vi "Actor Core.vi"(8 "error in":errorcluster, 11 "Philosopher in":refnum<class "Philosopher.lvclass">) -> (0 "error out":errorcluster, 3 "Philosopher out":refnum<class "Actor.lvclass">)   [LabVIEW 2023, in "Philosopher.lvlib" / "Philosopher.lvclass"]
doc: "(<B>Filename</B>: Actor Framework.lvlib:Actor.lvclass:Actor Core.vi)\n\nReceives messages to the actor, reacts to them, and initiates any error handling that may shut the actor down.\n\nDescendant classes may override this VI to append parallel tasks for the actor to complete while it handles messages. Overrides use the Call Parent Method node."
uses:
  Philosopher.lvclass
  C:/Program Files (x86)/National Instruments/LabVIEW 2023/vi.lib/ActorFramework/Actor/Actor.lvclass
  <vilib>/ActorFramework/Actor/Actor.lvclass
  State Picture.ctl
  Philosopher Statechart.lvsc/Inputs.ctl
  <vilib>/ActorFramework/Message Enqueuer/Message Enqueuer.lvclass
  Philosopher Statechart.lvsc/Trigger.ctl
  Philosopher.lvclass/Philosopher.ctl
  <vilib>/ActorFramework/Actor/Actor.lvclass/Actor.ctl
  <vilib>/ActorFramework/Message Enqueuer/Message Enqueuer.lvclass/Message Enqueuer.ctl
  <vilib>/Statechart/Common/IntGuid.ctl
  <vilib>/Statechart/Common/DbgID.ctl
  Philosopher Statechart.lvsc/StatechartState.ctl
  Philosopher Statechart.lvsc/State.ctl
  031f544c-a229-44b1-b513-832e3cf1e2d7.vi
  <vilib>/ActorFramework/Message Enqueuer/Init from Existing Queue.vi
  Philosopher Statechart.lvsc/CompanionDiagram.vi/26/SC Main.vi
  <vilib>/Statechart/Infrastructure/RTStatechart/RunTime SCN.xnode
  Philosopher Statechart.lvsc/Outputs.ctl
  Philosopher Statechart.lvsc
  <vilib>/Statechart/Nodes/EventFiring/NI_SC_EventFiringNode.xnode
  <vilib>/Statechart/Common/NI_SC_LVSCCommonFiles.lvlib
panel:
  out "Diagram Display":picture
  out "ID":i32
  out "State Picture":T1=3
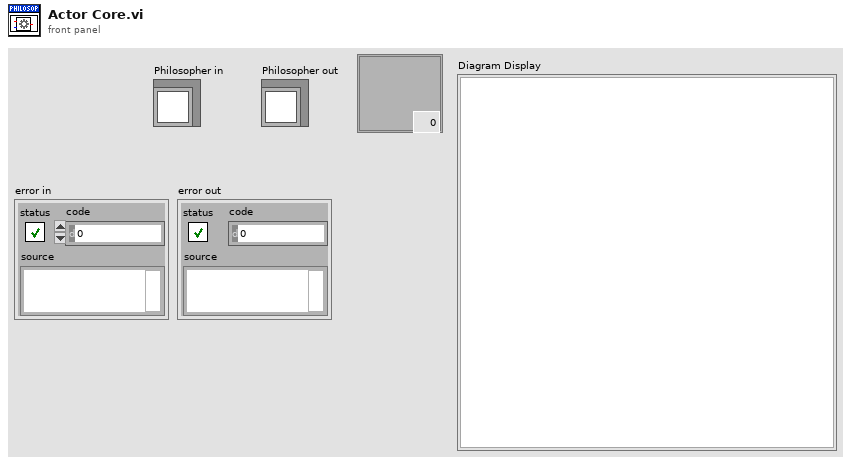
[diagram p1: front panel]
types:
  T1 = typedef "Philosopher.lvlib/Philosopher.lvclass/State Picture.ctl" = u16
  T2 = typedef "Philosopher.lvlib/Philosopher Statechart.lvsc/Trigger.ctl" = enum16{"NULL", "TIMEOUT", "EXIT", "EAT"}
  T3 = typedef "Philosopher.lvlib/Philosopher Statechart.lvsc/Inputs.ctl" = cluster{"Self Enqueuer":refnum<class "Message Enqueuer.lvclass">, "Philosopher ID":i32, "Caller Enqueuer":refnum<class "Message Enqueuer.lvclass">}
  T4 = typedef "Rendezvous RefNum" = refnum<k1>
  T5 = typedef "NI_SC_LVSCCommonFiles.lvlib/IntGuid.ctl" = cluster{"Data1":u32, "Data2":u16, "Data3":u16, "Data4":u8, "Data5":u8, "Data6":u8, "Data11":u8, "Data9":u8, "Data10":u8, "Data8":u8, "Data7":u8}
  T6 = typedef "NI_SC_LVSCCommonFiles.lvlib/DbgID.ctl" = cluster{"VIRef":u32, "IntGUID":T5}
  T7 = typedef "Philosopher.lvlib/Philosopher Statechart.lvsc/Outputs.ctl" = enum16{"thinking", "hungry", "eating"}
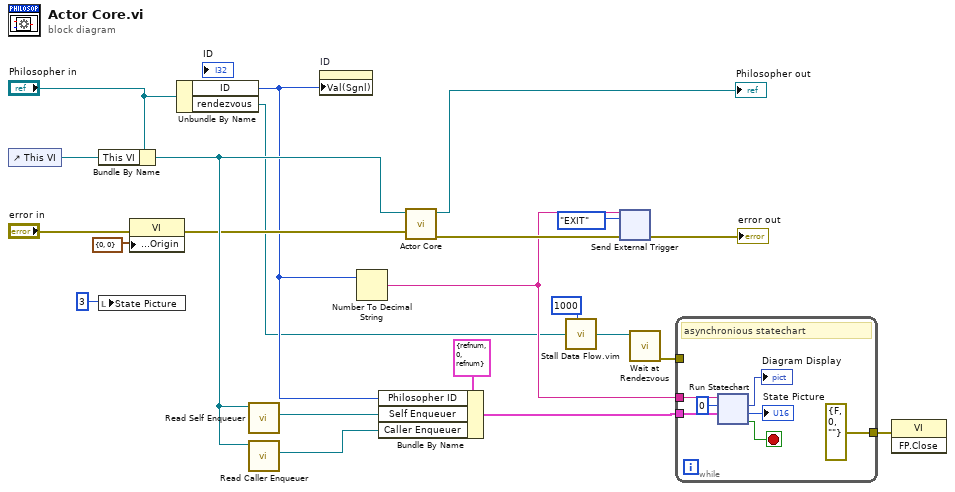
[diagram p0: block diagram]
diagram:
  n1 = control-ref of="This VI"() -> (w20:refnum<vi>)
  n2 = Bundle By Name(cluster="Philosopher in", "This VI"=w20) -> (w13:refnum<class "Philosopher.lvclass">)
  n3 = local write "State Picture"(T1 3 ("State Picture")) -> ()
  n4 = property class="VI"(error in="error in", "Front Panel Window:Origin"=cluster{"Horizontal":i16, "Vertical":i16} {"Horizontal"=0, "Vertical"=0}) -> (error out=w11:errorcluster)  [unwired: 1 in, 1 out]
  n5 = Unbundle By Name("Philosopher in") -> ("ID"=w5:i32, "rendezvous"=w3:T4)
  n6 = call <vilib>:"Read Self Enqueuer.vi"("Actor"=w13) -> ("Self Enqueuer"=w15:refnum<class "Message Enqueuer.lvclass">)  [unwired: 10 in]
  n7 = call <vilib>:"Read Caller Enqueuer.vi"("Actor"=w13) -> ("Caller Enqueuer"=w14:refnum<class "Message Enqueuer.lvclass">)  [unwired: 10 in]
  n8 = property on="ID" class="DigNum (strict)"("Val(Sgnl)"=w5) -> ()  [unwired: 2 in, 2 out]
  n9 = Number To Decimal String(number=w5) -> (decimal integer string=w8:string)  [unwired: 1 in]
  n10 = Bundle By Name(cluster=T3 {"Self Enqueuer"=refnum, "Philosopher ID"=0, "Caller Enqueuer"=refnum} ("Inputs"), "Philosopher ID"=w5, "Self Enqueuer"=w15, "Caller Enqueuer"=w14) -> (w16:T3)
  n11 = call-parent "Actor Core.vi"("error in"=w11, "Actor in"=w13) -> ("error out"=w10:errorcluster, "Actor out"=→"Philosopher out":refnum<class "Actor.lvclass">)  [unwired: 8 in]
  n12 = call "Stall Data Flow.vim"("value in"=w3, "milliseconds to wait"=u32 1000) -> ("value out"=w2:T4)  [unwired: 1 out]
  n13 = xnode "Send External Trigger"("Instance Name"=w8, "Trigger"=Trigger."EXIT", "error in (no error)"=w10) -> ("error out"=→"error out":errorcluster)  [unwired: 1 out]
  n14 = call <vilib>:"Wait at Rendezvous.vi"("rendezvous"=w2) -> ("error out"=w4:errorcluster)  [unwired: 4 in, 2 out]
  n15 = while {
    tunnel: w8 -> [w29]
    tunnel: w16 -> [w28]
    tunnel: [errorcluster {"status"=FALSE, "code"=0, "source"=""} ("error in (no error)")] -> w6
    tunnel: w4 -> [_]
    stop <- w27 stop-if-true
    # "asynchronious statechart"
    n16 = xnode "Run Statechart"("Inputs"=w28, "Instance Name"=w29, "Diagram Display Index"=u16 0) -> ("Terminated?"=w27:bool, "Outputs"=→"State Picture":T7, "Diagram Display"=→"Diagram Display":picture)  [unwired: 1 in, 1 out]
  }
  n17 = invoke on="Invoke Node" class="VI" method="FP.Close"(error in=w6) -> ()  [unwired: 2 in, 3 out]
